vi "Generate New Overlay.vi"(4 "Pixellate":bool, 6 "Label?":bool, 8 "error in":errorcluster, 10 "Lithography Data":T2(array[cluster]), 11 "BigMAQ in":refnum<class "BigMAQ.lvclass">) -> (0 "error out":errorcluster, 3 "BigMAQ out":refnum<class "BigMAQ.lvclass">)   [LabVIEW 2019, in "BigMAQ.lvclass"]
uses:
  BigMAQ.lvclass
  <userlib>/LevyLab/Relay Box/Typedefs/Resistor--enum.ctl
  BigMAQ.lvclass/BigMAQ.ctl
  <userlib>/LevyLab/Relay Box/Relay-Box.lvclass
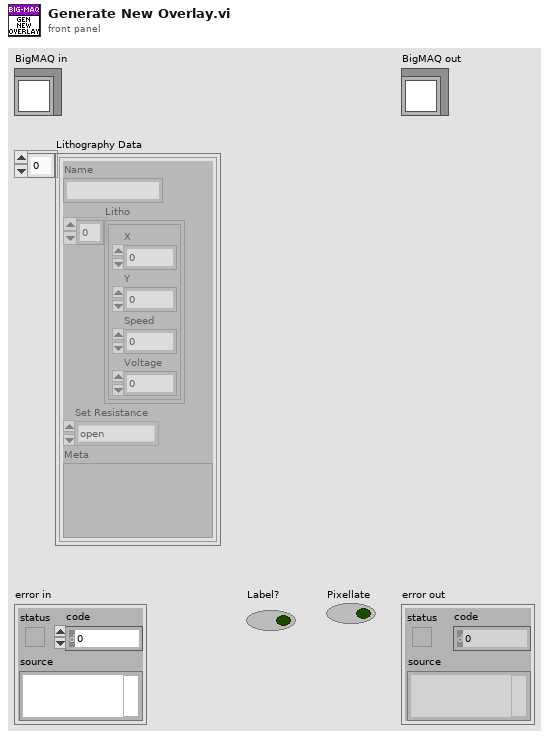
[diagram p1: front panel]
types:
  T1 = typedef "Relay-Box.lvclass/Resistor--enum.ctl" = enum16{"open", "discharge tip", "0 ohms", "100k ohm", "10M ohm", "1G ohm"}
  T2 = cluster{"Name":string, "Litho":cluster{"X":dbl, "Y":dbl, "Speed":dbl, "Voltage":dbl}[], "Set Resistance":T1, "Meta":variant}[]
  T3 = typedef "IMAQ Image.ctl" = refnum<image>
  T4 = typedef "BigMAQ.lvclass/Overlay.ctl" = cluster{"Name":string, "Data":cluster{"Points":cluster{"X":dbl, "Y":dbl}[], "Voltages":dbl[]}}
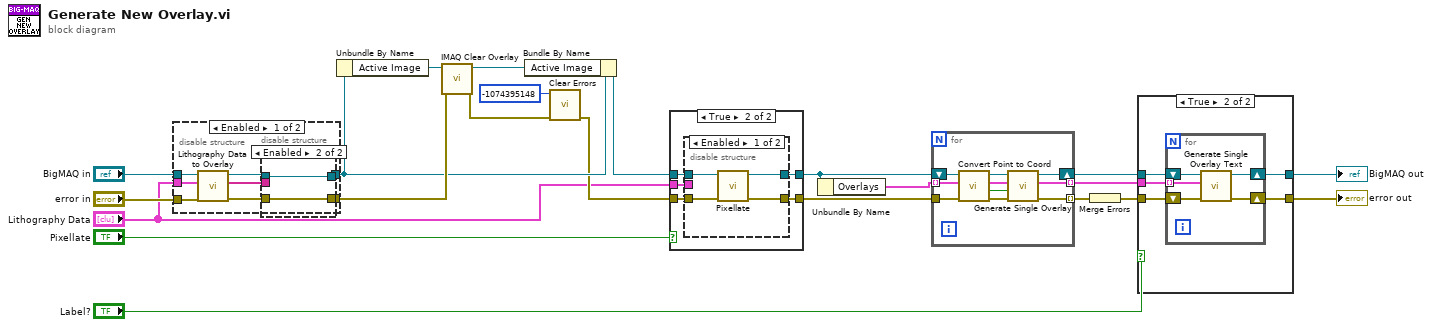
[diagram p0: block diagram]
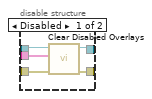
[diagram p2: hidden frame]
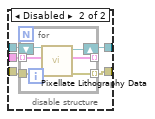
[diagram p5: hidden frame]
diagram:
  n1 = disable-structure shown="Enabled" {
    disable-tunnel: "BigMAQ in" -> [w30 w39]
    disable-tunnel: "error in" -> [w29 w38]
    disable-tunnel: [w25 w38] -> w9
    disable-tunnel: [w24 w39] -> w8
    disable-tunnel: "Lithography Data" -> [w23 _]
    frame Enabled {
      n2 = call "Lithography Data to Overlay.vi"("error in"=w29, "Lithography Data"=w23, "BigMAQ in"=w30) -> ("error out"=w27:errorcluster, "Disabled Overlays"=w26:string[], "BigMAQ out"=w28:refnum<class "BigMAQ.lvclass">)  [unwired: 6 in]
      n3 = disable-structure shown="Enabled" {
        disable-tunnel: w28 -> [w35 w37]
        disable-tunnel: w27 -> [w34 w36]
        disable-tunnel: w26 -> [w33 _]
        disable-tunnel: [w32 w36] -> w25
        disable-tunnel: [w31 w37] -> w24
        frame Disabled {
          n4 = call "Clear Disabled Overlays.vi"("error in"=w34, "Disabled Overlays"=w33, "BigMAQ in"=w35) -> ("error out"=w32:errorcluster, "BigMAQ out"=w31:refnum<class "BigMAQ.lvclass">)  [unwired: 7 in]
        }
        frame Enabled {
        }
      }
    }
    frame Disabled {
    }
  }
  n5 = Unbundle By Name(w8) -> ("Active Image"=w11:T3)
  n6 = call "IMAQ Clear Overlay"("error in (no error)"=w9, "Image"=w11) -> ("error out"=w6:errorcluster, "Image Out"=w10:T3)  [unwired: 8 in]
  n7 = Bundle By Name(cluster=w8, "Active Image"=w10) -> (w12:refnum<class "BigMAQ.lvclass">)
  n8 = call <vilib>:"Clear Errors.vi"("error in (no error)"=w6, "specific error code to clear (0: all)"=-1074395148) -> ("error out"=w5:errorcluster)  [unwired: 4 in, 1 out]
  n9 = case shown="True" "Pixellate" {
    tunnel: [_ w45] -> w13
    tunnel: [w40 w44] -> w2
    tunnel: w12 -> [w40 w43]
    tunnel: w5 -> [_ w42]
    tunnel: "Lithography Data" -> [_ w41]
    frame False {
    }
    frame True {
      n10 = disable-structure shown="Enabled" {
        disable-tunnel: [w49 w51] -> w45
        disable-tunnel: [w48 w53] -> w44
        disable-tunnel: w43 -> [w47 w54]
        disable-tunnel: w42 -> [w46 w52]
        disable-tunnel: w41 -> [_ w50]
        frame Enabled {
          n11 = call "Pixellate.vi"("error in"=w46, "BigMAQ in"=w47) -> ("error out"=w49:errorcluster, "BigMAQ out"=w48:refnum<class "BigMAQ.lvclass">)  [unwired: 8 in]
        }
        frame Disabled {
          n12 = for {
            shift-right: [w59] -> w53
            shift-left: w54 -> [w60]
            tunnel: w52 -> [w58]
            tunnel: [w57] -> w51 mode=indexing
            tunnel: [w56] -> _ mode=indexing
            tunnel: w50 -> [w55] mode=indexing
            n13 = call "Pixellate Lithography Data.vi"("error in"=w58, "Lithography Data"=w55, "BigMAQ in"=w60) -> ("error out"=w57:errorcluster, "Array"=w56:T4[], "BigMAQ out"=w59:refnum<class "BigMAQ.lvclass">)  [unwired: 6 in]
          }
        }
      }
    }
  }
  n14 = Unbundle By Name(w2) -> ("Overlays"=w1:T4[])
  n15 = for {
    tunnel: w1 -> [w64] mode=indexing
    tunnel: w13 -> [w62]
    tunnel: [w69] -> w22 mode=indexing
    shift-right: [w70] -> w19
    shift-left: w2 -> [w67]
    tunnel: [w68] -> w14 mode=indexing
    n16 = call "Convert Point to Coord.vi"("error in"=w62, "Overlay"=w64, "BigMAQ in"=w67) -> ("error out"=w63:errorcluster, "Voltage Constant?"=w61:bool, "output cluster"=w65:T4, "BigMAQ out"=w66:refnum<class "BigMAQ.lvclass">)  [unwired: 5 in]
    n17 = call "Generate Single Overlay.vi"("error in"=w63, "Single Color"=w61, "Overlay"=w65, "BigMAQ in"=w66) -> ("error out"=w69:errorcluster, "Overlay Out"=w68:T4, "BigMAQ out"=w70:refnum<class "BigMAQ.lvclass">)  [unwired: 5 in]
  }
  n18 = Merge Errors(w22) -> (w17:errorcluster)
  n19 = case shown="True" "Label?" {
    tunnel: w19 -> [w72 w77]
    tunnel: [w72 w76] -> w18
    tunnel: w17 -> [w71 w75]
    tunnel: [w71 w74] -> w16
    tunnel: w14 -> [_ w73]
    frame False {
    }
    frame True {
      n20 = for {
        tunnel: w73 -> [w78] mode=indexing
        shift-right: [w81] -> w76
        shift-left: w77 -> [w82]
        shift-right: [w79] -> w74
        shift-left: w75 -> [w80]
        n21 = call "Generate Single Overlay Text.vi"("error in"=w80, "Overlay"=w78, "BigMAQ in"=w82) -> ("error out"=w79:errorcluster, "BigMAQ out"=w81:refnum<class "BigMAQ.lvclass">)  [unwired: 7 in]
      }
    }
  }
  "error out" <- w16
  "BigMAQ out" <- w18
